vi "总磷总氮启动参数对话框.vi"() -> (2 "确认":bool, 3 "元素":cluster{"命令":string, "data":variant})   [LabVIEW 2016, in "斯坦道总氮.lvlib"]
panel:
  out "标液值":dbl caption="标液值："
  in  "取消":bool
  in  "确定":bool
  in  "量程切换":u16(ring)=2 items=["H", "L", "AUTO"]
  in  "站号":u16(ring)=1 items=["氨氮"=3, "总磷"=1]
  in  "控制命令":T1(ring)
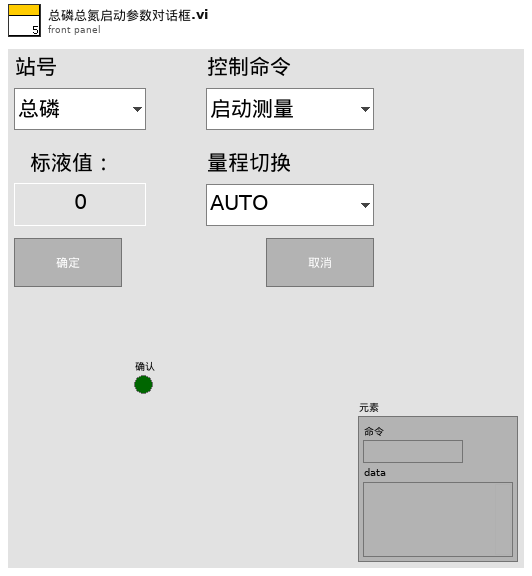
[diagram p1: front panel]
types:
  T1 = enum16{"启动测量", "标样核查", "零点核查", "跨度核查", "空白测试", "平行样测试", "加标回收", "空白校准", "标样校准", "初始化（清洗）", "停止测试", "仪器重启", "校时", "模式设置", "测量间隔设置"}
  T2 = cluster{"站号":u16, "量程切换":enum32{"H", "L", "AUTO"}, "控制命令":enum16{"启动测量", "标样核查", "零点核查", "跨度核查", "空白测试", "平行样测试", "加标回收", "空白校准", "标样校准", "初始化（清洗）", "停止测试", "仪器重启", "校时", "模式设置", "测量间隔设置", "盲样测试"}, "模式设置":enum16{"待机", "连续模式", "周期模式", "定点模式", "受控模式", "手动模式"}, "测量间隔":u16}
  T3 = cluster{"总磷跨度值":dbl, "总磷零点标准液浓度":dbl, "总磷跨度标准液浓度":dbl, "总磷标准液标准浓度":dbl, "总氮跨度值":dbl, "总氮零点标准液浓度":dbl, "总氮跨度标准液浓度":dbl, "总氮标准液标准浓度":dbl, "COD跨度值":dbl, "COD零点标准液浓度":dbl, "COD跨度标准液浓度":dbl, "COD标准液标准浓度":dbl, "氨氮跨度值":dbl, "氨氮零点标准液浓度":dbl, "氨氮跨度标准液浓度":dbl, "氨氮标准液标准浓度":dbl}
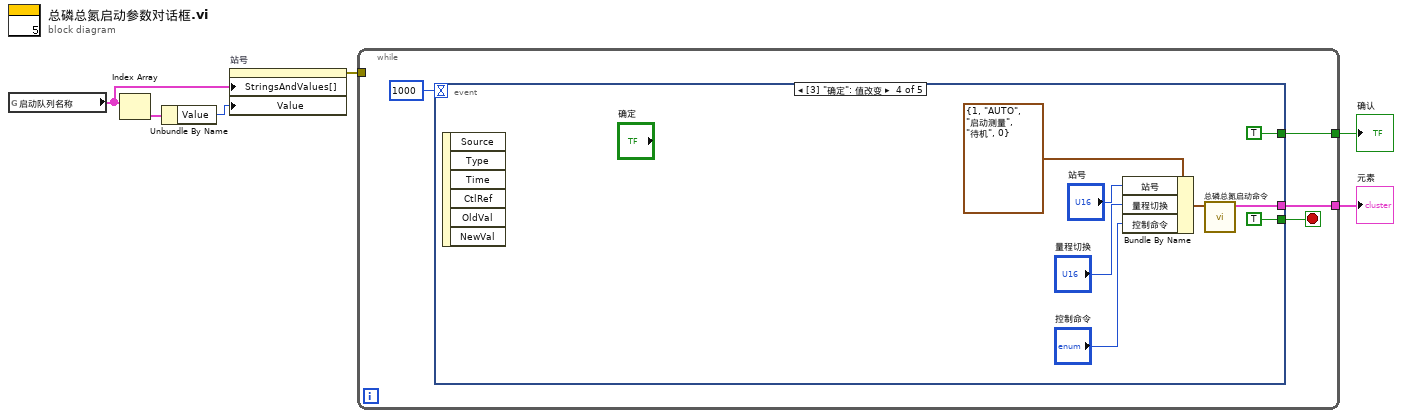
[diagram p0: block diagram]
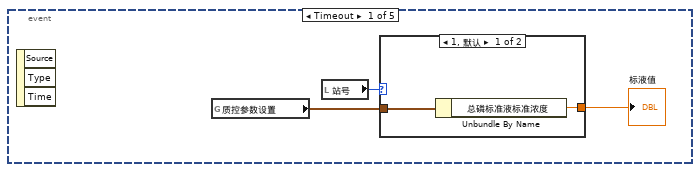
[diagram p2: hidden frame]
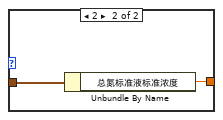
[diagram p3: hidden frame]
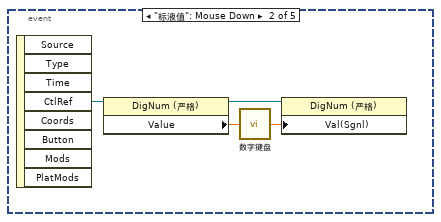
[diagram p4: hidden frame]
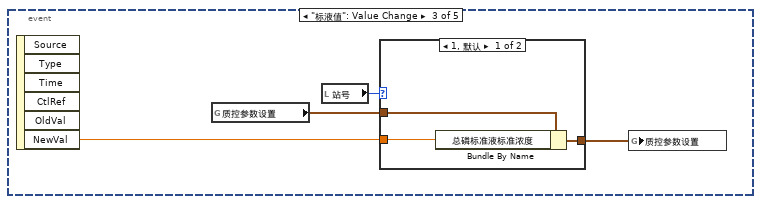
[diagram p5: hidden frame]
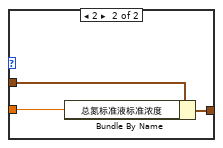
[diagram p6: hidden frame]
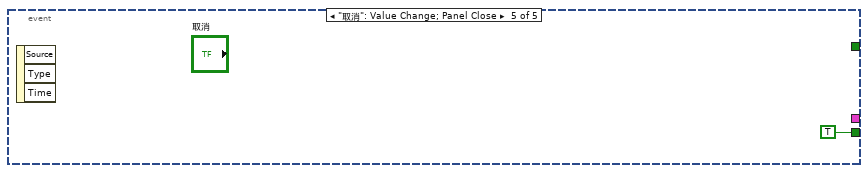
[diagram p7: hidden frame]
diagram:
  n1 = global read "VAR总磷总氮全局变量.vi" "启动队列名称"() -> (w1:cluster{"String":string, "Value":u16}[])
  n2 = Index Array(array=w1) -> (element=w4:cluster{"String":string, "Value":u16})  [unwired: 1 in]
  n3 = Unbundle By Name(w4) -> ("Value"=w3:u16)
  n4 = property on="站号" class="Ring (严格)"("StringsAndValues[]"=w1, "Value"=w3) -> (error out=w2:errorcluster)  [unwired: 2 in, 1 out]
  n5 = while {
    tunnel: [w8] -> w6
    tunnel: [w7] -> w5
    tunnel: w2 -> [_]
    stop <- w10 stop-if-true
    n6 = event shown="[3] \"确定\": 值改变" {
      selector: _ -> [_ _ _ _ _]
      dyn-events: _ -> [_ _ _ _ _]
      timeout: 1000 -> [_ _ _ _ _]
      tunnel: [_ _ _ TRUE TRUE] -> w10
      tunnel: [_ _ _ TRUE _] -> w8
      tunnel: [_ _ _ w37 _] -> w7
      event Timeout {
        n7 = event-data() -> ()  [unwired: 1 in, 3 out]
        n8 = global read "总磷总氮断电保存全局变量.vi" "质控参数设置"() -> (w13:T3)
        n9 = local read "站号"() -> (w12:u16)
        n10 = case shown="1, 默认" w12 {
          tunnel: w13 -> [w15 w17]
          tunnel: [w14 w16] -> w11
          frame 1, Default {
            n11 = Unbundle By Name(w15) -> ("总磷标准液标准浓度"=w14:dbl)
          }
          frame 2 {
            n12 = Unbundle By Name(w17) -> ("总氮标准液标准浓度"=w16:dbl)
          }
        }
        "标液值" <- w11
      }
      event "标液值": Mouse Down {
        n13 = event-data() -> ("CtlRef"=w21:refnum<vi>)  [unwired: 1 in, 7 out]
        n14 = property class="DigNum (严格)"(reference=w21) -> (reference out=w18:refnum<vi>, "Value"=w20:dbl)  [unwired: 1 in, 1 out]
        n15 = call "数字键盘.vi"("OldNumber"=w20) -> ("NewNumber"=w19:dbl)
        n16 = property class="DigNum (严格)"(reference=w18, "Val(Sgnl)"=w19) -> ()  [unwired: 1 in, 2 out]
      }
      event "标液值": Value Change {
        n17 = event-data() -> ("NewVal"=w23:dbl)  [unwired: 1 in, 5 out]
        n18 = global read "总磷总氮断电保存全局变量.vi" "质控参数设置"() -> (w24:T3)
        n19 = local read "站号"() -> (w25:u16)
        n20 = case shown="1, 默认" w25 {
          tunnel: w24 -> [w28 w31]
          tunnel: [w26 w29] -> w22
          tunnel: w23 -> [w27 w30]
          frame 1, Default {
            n21 = Bundle By Name(cluster=w28, "总磷标准液标准浓度"=w27) -> (w26:T3)
          }
          frame 2 {
            n22 = Bundle By Name(cluster=w31, "总氮标准液标准浓度"=w30) -> (w29:T3)
          }
        }
        n23 = global write "总磷总氮断电保存全局变量.vi" "质控参数设置"(w22) -> ()
      }
      event "确定": Value Change {
        n24 = event-data() -> ()  [unwired: 1 in, 6 out]
        n25 = Bundle By Name(cluster=T2 {"站号"=1, "量程切换"=enum."AUTO", "控制命令"=enum."启动测量", "模式设置"=enum."待机", "测量间隔"=0} ("参数"), "站号"="站号", "量程切换"="量程切换", "控制命令"="控制命令") -> (w35:T2)
        n26 = call "总磷总氮启动命令.vi"("参数"=w35) -> ("启动命令"=w37:cluster{"命令":string, "data":variant})  [unwired: 10 in]
      }
      event "取消": Value Change; Panel Close {
        n27 = event-data() -> ()  [unwired: 1 in, 3 out]
      }
    }
  }
  "元素" <- w5
  "确认" <- w6
